vi "Add.vi"(8 "error in (no error)":errorcluster, 9 "Project":refnum<vi>, 10 "IB_Destination.lvclass":refnum<class "IB_Destination.lvclass">, 11 "IB_Tree_Item_Proj_File in":refnum<class "IB_Tree_Item_Proj_File.lvclass">) -> (0 "error out":errorcluster, 1 "updated?":bool, 2 "IB_Source.lvclass":refnum<class "IB_Source.lvclass">, 3 "IB_Tree_Item_Proj_File out":refnum<class "IB_Tree_Item_Proj_File.lvclass">)   [LabVIEW 2020, in "IB_Tree_Item_Proj_File.lvclass"]
uses:
  <vilib>/AppBuilder/IB_Classes/Tree_Item_Proj_File/IB_Tree_Item_Proj_File.lvclass
  <vilib>/AppBuilder/IB_Classes/Tree_Item_Proj_File/IB_Tree_Item_Proj_File.lvclass/IB_Tree_Item_Proj_File.ctl
  <vilib>/AppBuilder/IB_Classes/Source/IB_Source.lvclass
  <vilib>/AppBuilder/IB_Classes/Destination/IB_Destination.lvclass
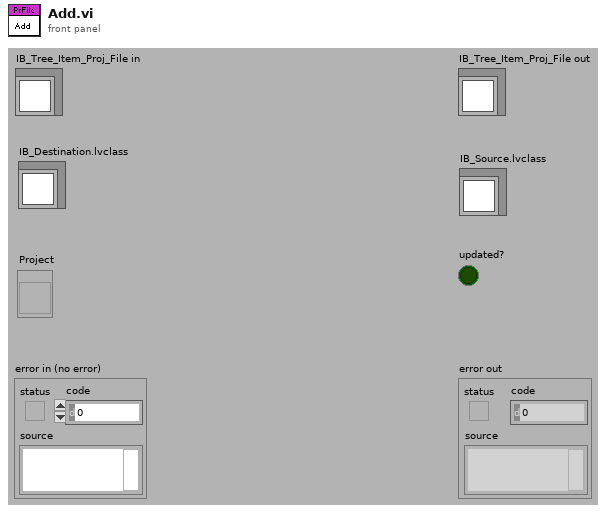
[diagram p1: front panel]
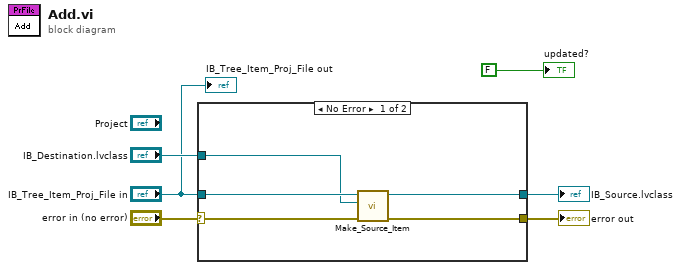
[diagram p0: block diagram]
diagram:
  n1 = case shown="No Error" "error in (no error)" {
    selector: "error in (no error)" -> [w11 w12]
    tunnel: [w9 _] -> w6
    tunnel: "IB_Tree_Item_Proj_File in" -> [w10 _]
    tunnel: [w8 w12] -> w5
    tunnel: "IB_Destination.lvclass" -> [w7 _]
    frame No Error {
      n2 = call-dynamic "Make_Source_Item.vi"("error in (no error)"=w11, "IB_Destination.lvclass"=w7, "IB_Tree_Item_Proj_File in"=w10) -> ("error out"=w8:errorcluster, "IB_Source.lvclass"=w9:refnum<class "IB_Source.lvclass">)  [unwired: 7 in]
    }
    frame Error {
    }
  }
  "error out" <- w5
  "IB_Source.lvclass" <- w6
  "IB_Tree_Item_Proj_File out" <- "IB_Tree_Item_Proj_File in"
  "updated?" <- FALSE
